vi "Configure Target Weight.vi"(8 "error in (no error)":errorcluster, 10 "Target Weight [g]":dbl, 11 "VISA resource name":refnum<visa-resource-name>) -> (0 "error out":errorcluster, 3 "VISA resource name out":refnum<visa-resource-name>)   [LabVIEW 2017, in "RadWag balances and scales.lvlib"]
doc: "Sets target mass in dosing mode.\nThis VI works properly when balance works in dosing mode. (To configure work mode use Utility -> Set Operating Mode)"
uses:
  <instrlib>/Prev/RadWag Continuous Read Folder/RadWag balances and scales.lvlib
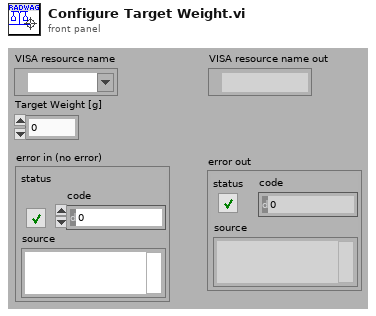
[diagram p1: front panel]
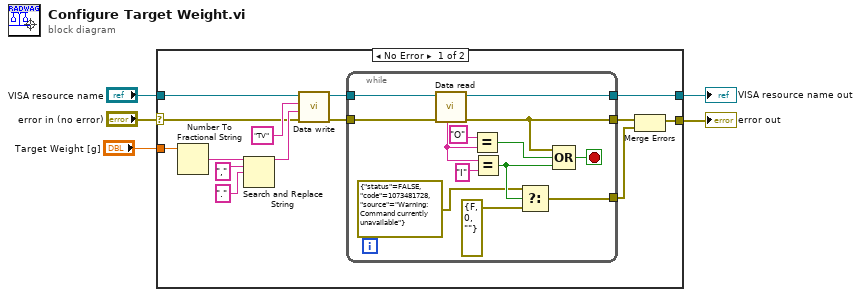
[diagram p0: block diagram]
diagram:
  n1 = case shown="No Error" "error in (no error)" {
    selector: "error in (no error)" -> [w9 w33]
    tunnel: "VISA resource name" -> [w19 w34]
    tunnel: [w16 w34] -> w4
    tunnel: "Target Weight [g]" -> [w14 _]
    tunnel: [w7 w33] -> w1
    frame No Error {
      n2 = Number To Fractional String(number=w14) -> (F-format string=w13:string)  [unwired: 3 in]
      n3 = Search and Replace String(input string=w13, search string=",", replace string="." ("replace string (\"\")")) -> (result string=w10:string)  [unwired: 5 in, 3 out]
      n4 = call <instrlib>:"Data write.vi"("error in (no error)"=w9, "Parameter"=w10, "ID"="TV", "VISA resource name"=w19) -> ("error out"=w17:errorcluster, "VISA resource name out"=w18:refnum<visa-resource-name>)  [unwired: 6 in]
      n5 = while {
        tunnel: w18 -> [w32]
        tunnel: w17 -> [w31]
        tunnel: [w30] -> w16
        tunnel: [w26] -> w8
        tunnel: [w21] -> w6
        stop <- w25 stop-if-true
        n6 = call <instrlib>:"Data read.vi"("error in (no error)"=w31, "VISA resource name"=w32) -> ("error out"=w26:errorcluster, "VISA resource name out"=w30:refnum<visa-resource-name>, "Status"=w29:string)  [unwired: 3 in, 4 out]
        n7 = Equal?(x="O", y=w29) -> (x = y?=w24:bool)
        n8 = Equal?(x=w29, y="I") -> (x = y?=w23:bool)
        n9 = Select(t=errorcluster {"status"=FALSE, "code"=1073481728, "source"="Warning: Command currently unavailable"}, s=w23, f=errorcluster {"status"=FALSE, "code"=0, "source"=""} ("error constant")) -> (s? t:f=w21:errorcluster)
        n10 = Compound Arithmetic op=OR(w26, w24, w23) -> (w25:bool)
      }
      n11 = Merge Errors(w8, w6) -> (w7:errorcluster)
    }
    frame Error {
    }
  }
  "VISA resource name out" <- w4
  "error out" <- w1
